vi "Ctor.vi"(8 "error in (no error)":errorcluster, 11 "BoardArrayPanel in":refnum<class "BoardArrayPanel.lvclass">) -> (0 "error out":errorcluster, 3 "BoardArrayPanel out":refnum<class "BoardArrayPanel.lvclass">)   [LabVIEW 2020, in "PicoG-App.lvlib" / "BoardArrayPanel.lvclass"]
uses:
  BoardArrayPanel.lvclass
  <vilib>/IlluminatedG/IG OOPanel/OOPanel/ArrayPanel/ArrayPanel.lvclass
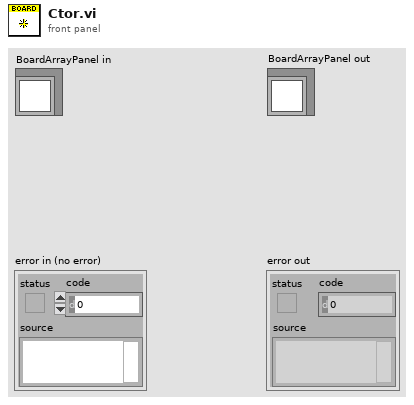
[diagram p1: front panel]
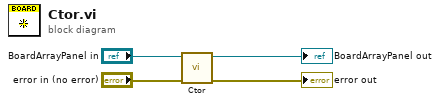
[diagram p0: block diagram]
diagram:
  n1 = call-parent "Ctor.vi"("error in (no error)"="error in (no error)", "ArrayPanel in"="BoardArrayPanel in") -> ("error out"=→"error out":errorcluster, "ArrayPanel out"=→"BoardArrayPanel out":refnum<class "BoardArrayPanel.lvclass">)  [unwired: 8 in]
